vi "Init.vi"(3 "Container State":T5, 4 "Previous State":variant, 5 "Previous Version":T4) -> (2 "Current State":T1={"SP_Source"={"connect"=FALSE, "SP_Source"=enum."initialize", "SP_Set"=0.0, "SP"=0.0}, "Write"=FALSE, "button state"=enum."init", "reset_timer"=FALSE, "load_timer"=FALSE, "Time"=0, "t ms"=0, "tick"=0, "scale maximum"=100.0})   [LabVIEW 2019, in "control.lvlib" / "SP_h1.xctl"]
uses:
  SP_h1.xctl
  State.ctl
  Heating/ctl/Y_source.ctl
  Y_controlState.ctl
  <vilib>/_xctls/Container State.ctl
  <vilib>/_xctls/Version.ctl
  <vilib>/_xctls/XControlSupport.lvlib
  Heating/Heating.lvlib
panel:
  in  "Default Indicator State":T1={"SP_Source"={"connect"=FALSE, "SP_Source"=enum."initialize", "SP_Set"=0.0, "SP"=0.0}, "Write"=FALSE, "button state"=enum."init", "reset_timer"=FALSE, "load_timer"=FALSE, "Time"=0, "t ms"=0, "tick"=0, "scale maximum"=100.0}
  in  "Default Control State":T1={"SP_Source"={"connect"=FALSE, "SP_Source"=enum."initialize", "SP_Set"=0.0, "SP"=0.0}, "Write"=FALSE, "button state"=enum."init", "reset_timer"=FALSE, "load_timer"=FALSE, "Time"=0, "t ms"=0, "tick"=0, "scale maximum"=100.0}
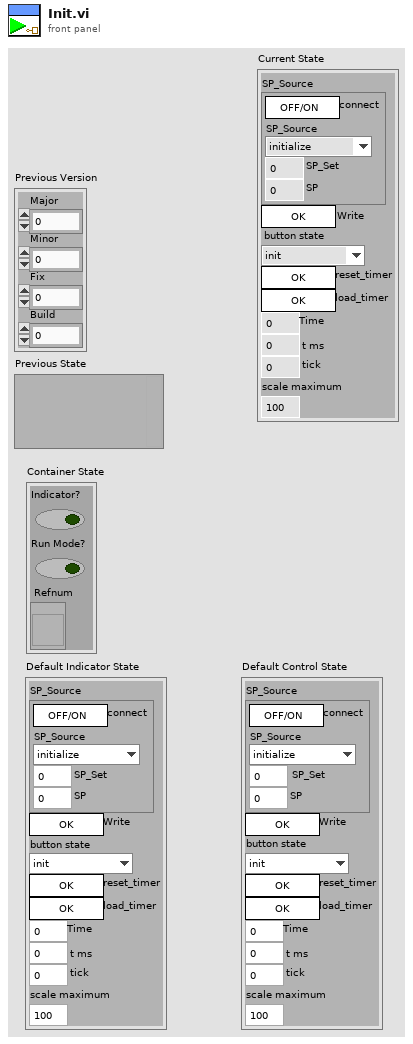
[diagram p1: front panel]
types:
  T1 = typedef "control.lvlib/SP_h1.xctl/State.ctl" = cluster{"SP_Source":cluster{"connect":bool, "SP_Source":T2, "SP_Set":dbl, "SP":dbl}, "Write":bool, "button state":T3, "reset_timer":bool, "load_timer":bool, "Time":u32, "t ms":u32, "tick":u32, "scale maximum":dbl}
  T2 = typedef "Heating.lvlib/Y_source.ctl" = enum8{"initialize", "local disabled", "local hand", "hand", "auto", "dist"}
  T3 = typedef "control.lvlib/SP_h1.xctl/Y_controlState.ctl" = enum16{"init", "not connect", "local disabled", "local hand", "hand", "value change", "auto", "dist"}
  T4 = typedef "XControlSupport.lvlib/Version.ctl" = cluster{"Major":u16, "Minor":u16, "Fix":u16, "Build":u16}
  T5 = typedef "XControlSupport.lvlib/Container State.ctl" = cluster{"Indicator?":bool, "Run Mode?":bool, " Refnum":refnum<vi>}
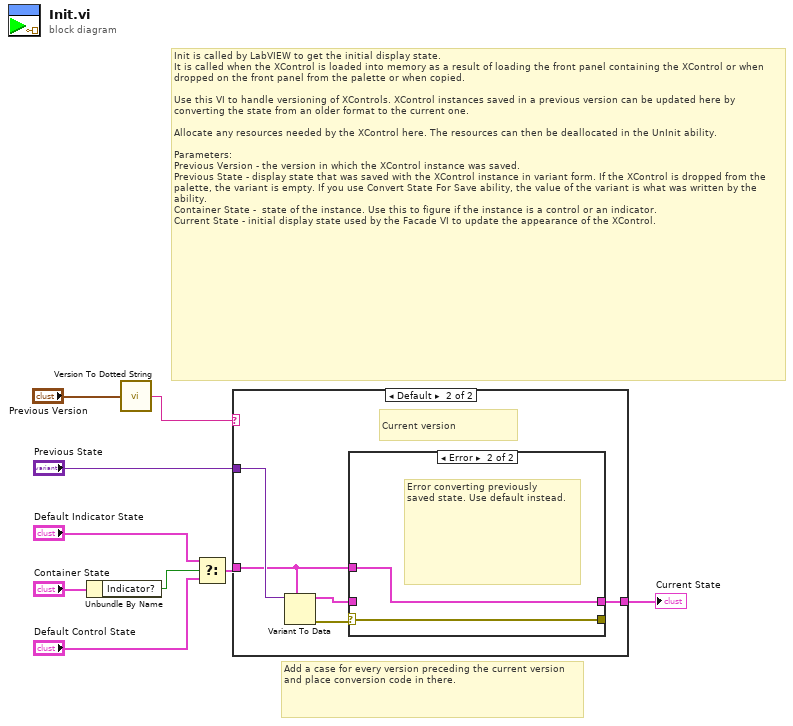
[diagram p0: block diagram]
diagram:
  # "Add a case for every version preceding the current version and place conversion code in there."
  # "Init is called by LabVIEW to get the initial display state.\nIt is called when the XControl is loaded into memory as a result of loading the front panel containing the XControl or when dropped on the front panel from the palette or when copied.\n\nUse this VI to handle versioning of XControls. XControl instances saved in a previous version can be updated here by converting the state from an older format to the current one.\n\nAllocate any resources needed by the XControl here. The resources can then be deallocated in the UnInit ability.\n\nParameters:\nPrevious Version - the version in which the XControl instance was saved.\nPrevious State - display state that was saved with the XControl instance in variant form. If the XControl is dropped from the palette, the variant is empty. If you use Convert State For Save ability, the value of the variant is what was written by the ability. \nContainer State -  state of the instance. Use this to figure if the instance is a control or an indicator.\nCurrent State - initial display state used by the Facade VI to update the appearance of the XControl."
  n1 = Unbundle By Name("Container State") -> ("Indicator?"=w4:bool)
  n2 = call <vilib>:"Version To Dotted String.vi"("Version"="Previous Version") -> ("String Version"=w1:string)
  n3 = Select(t="Default Indicator State", s=w4, f="Default Control State") -> (s? t:f=w3:T1)
  n4 = case shown="Default" w1 {
    tunnel: "Previous State" -> [_ w15]
    tunnel: [w10 w11] -> w8
    tunnel: w3 -> [w10 w12]
    frame "0.0.0.0" {
      # "Just created, use default state"
    }
    frame Default {
      # "Current version"
      n5 = Variant To Data(type=w12, Variant=w15) -> (data=w13:T1, error out=w14:errorcluster)  [unwired: 1 in]
      n6 = case shown="Error" w14 {
        selector: w14 -> [w17 w18]
        tunnel: w13 -> [w16 _]
        tunnel: [w16 w19] -> w11
        tunnel: w12 -> [_ w19]
        tunnel: [w17 w18] -> _
        frame No Error {
        }
        frame Error {
          # "Error converting previously \nsaved state. Use default instead."
        }
      }
    }
  }
  "Current State" <- w8
